vi "simulation_data.vi"() -> ()   [LabVIEW 2024]
uses:
  <vilib>/Utility/file.llb/Read Delimited Spreadsheet (string).vi
  <vilib>/ptbypt/NI_PtbyPt.lvlib
panel:
  out "double precision float":dbl
  out "XY Graph":cluster{dbl[], dbl[]}[](graph)
  in  "stop":bool
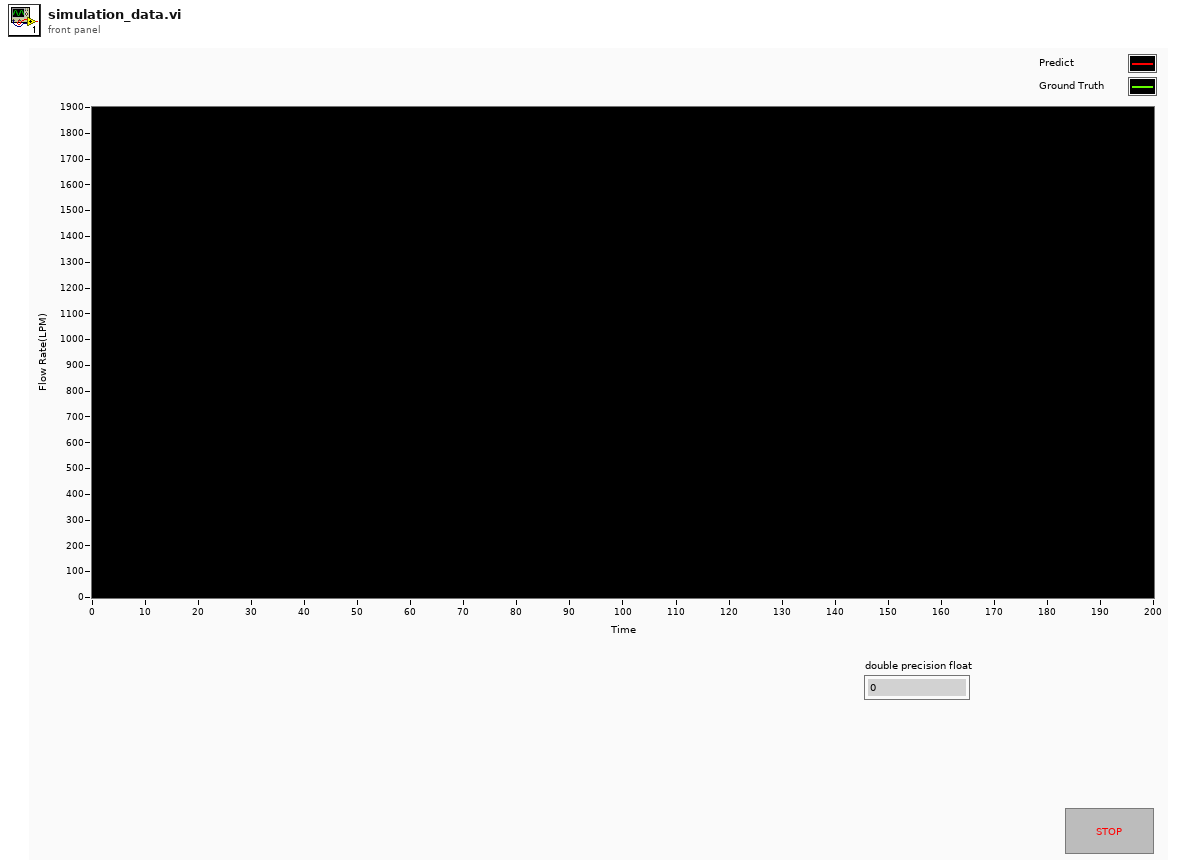
[diagram p1: front panel]
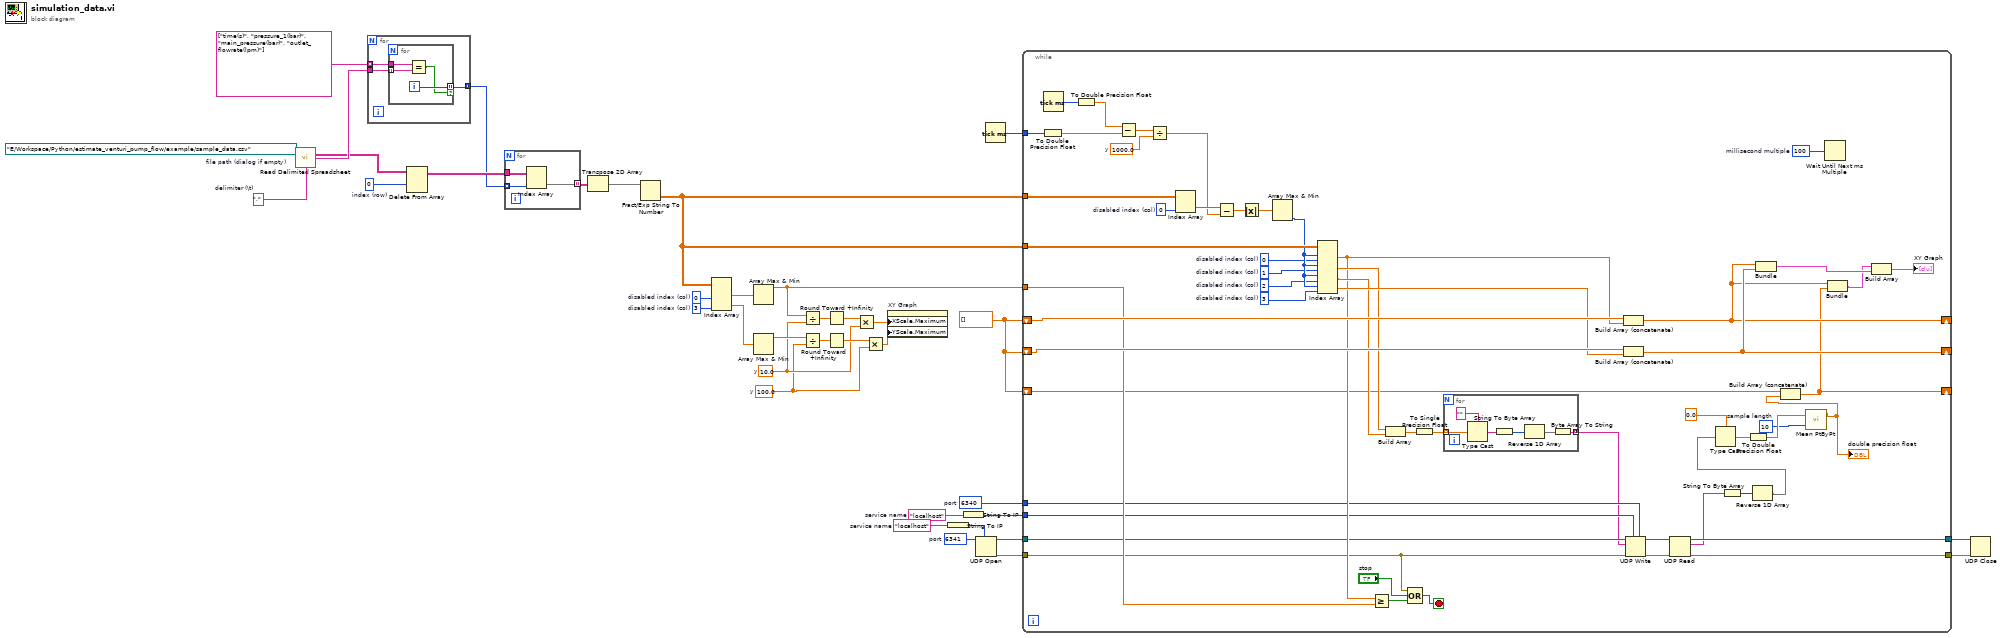
[diagram p0: block diagram]
diagram:
  w5 = "localhost"  # service name
  w1 = u16 6340  # port
  w8 = "localhost"  # service name
  w7 = u16 6341  # port
  w13 = 100.0  # y
  w16 = 10.0  # y
  w9 = dbl[] []
  w24 = 3  # disabled index (col)
  w25 = 0  # disabled index (col)
  w32 = 0  # index (row)
  w36 = ","  # delimiter (\t)
  w37 = path "E:/Workspace/Python/estimate_venturi_pump_flow/example/sample_data.csv"  # file path (dialog if empty)
  n1 = call-poly <vilib>:"Read Delimited Spreadsheet.vi"("file path (dialog if empty)"=w37, "delimiter (\\t)"=w36) -> ("all rows"=w33:string[][], "first row"=w35:string[])  [unwired: 8 in, 4 out]
  n2 = for {
    tunnel: w35 -> [w40]
    tunnel: string[] ["time(s)", "pressure_1(bar)", "main_pressure(bar)", "outlet_flowrate(lpm)"] -> [w39] mode=indexing
    tunnel: [w38] -> w30 mode=concatenating
    n3 = for {
      tunnel: w40 -> [w44] mode=indexing
      tunnel: w39 -> [w43]
      tunnel: [w42] -> w38 mode=indexing if=w41
      i -> [w42]
      n4 = Equal?(x=w43, y=w44) -> (x = y?=w41:bool)
    }
  }
  n5 = Delete From Array "Delete From Array"(array=w33, index (row)=w32) -> (array with subset deleted=w31:string[][])  [unwired: 2 in, 1 out]
  n6 = for {
    tunnel: w31 -> [w47]
    tunnel: w30 -> [w46] mode=indexing
    tunnel: [w45] -> w29 mode=indexing
    n7 = Index Array "Index Array"(array=w47, index (col)=w46) -> (element=w45:string[])  [unwired: 1 in]
  }
  n8 = Transpose 2D Array(2D array=w29) -> (transposed array=w28:string[][])
  n9 = Fract/Exp String To Number(string=w28) -> (number=w26:dbl[][])  [unwired: 3 in, 1 out]
  n10 = Index Array "Index Array"(array=w26, index (col) #1=w25, index (col) #2=w24) -> (element #1=w23:dbl[], element #2=w22:dbl[])  [unwired: 2 in]
  n11 = Array Max & Min(array=w23) -> (max value=w12:dbl)  [unwired: 3 out]
  n12 = Array Max & Min(array=w22) -> (max value=w21:dbl)  [unwired: 3 out]
  n13 = Divide(x=w12, y=w16) -> (x/y=w20:dbl)
  n14 = Divide(x=w21, y=w13) -> (x/y=w19:dbl)
  n15 = Round Toward +Infinity(x=w20) -> (ceil(x): smallest int >= x=w18:dbl)
  n16 = Round Toward +Infinity(x=w19) -> (ceil(x): smallest int >= x=w17:dbl)
  n17 = Multiply(x=w18, y=w16) -> (x*y=w15:dbl)
  n18 = Multiply(x=w17, y=w13) -> (x*y=w14:dbl)
  n19 = property on="XY Graph" class="XYGraph (strict)"("XScale.Maximum"=w15, "YScale.Maximum"=w14) -> ()  [unwired: 2 in, 2 out]
  n20 = String To IP(1:w8) -> (0:w6:u32)
  n21 = String To IP(1:w5) -> (0:w2:u32)
  n22 = UDP Open(7:w6, 11:w7) -> (port=w4:refnum<k16>, 0:w3:errorcluster)  [unwired: 3 in, 1 out]
  n23 = Tick Count (ms)() -> (millisecond timer value=w27:u32)
  n24 = while {
    tunnel: w27 -> [w100]
    tunnel: w26 -> [w95]
    tunnel: w26 -> [w89]
    shift-right: [w66] -> _
    shift-left: w9 -> [w82]
    shift-right: [w67] -> _
    shift-left: w9 -> [w81]
    tunnel: w12 -> [w73]
    tunnel: w4 -> [w71]
    tunnel: w3 -> [w56]
    tunnel: [w62] -> w11
    tunnel: [w61] -> w10
    shift-right: [w65] -> _
    shift-left: w9 -> [w69]
    tunnel: w2 -> [w58]
    tunnel: w1 -> [w57]
    stop <- w75 stop-if-true
    w49 = 10  # sample length
    w83 = 3  # disabled index (col)
    w84 = 2  # disabled index (col)
    w85 = 1  # disabled index (col)
    w86 = 0  # disabled index (col)
    w94 = 0  # disabled index (col)
    w96 = 1000.0  # y
    w102 = u32 100  # millisecond multiple
    n25 = To Double Precision Float(number=w100) -> (double precision float=w98:dbl)
    n26 = Tick Count (ms)() -> (millisecond timer value=w101:u32)
    n27 = To Double Precision Float(number=w101) -> (double precision float=w97:dbl)
    n28 = Subtract(x=w97, y=w98) -> (x-y=w99:dbl)
    n29 = Divide(x=w99, y=w96) -> (x/y=w92:dbl)
    n30 = Index Array "Index Array"(array=w95, index (col)=w94) -> (element=w93:dbl[])  [unwired: 1 in]
    n31 = Subtract(x=w93, y=w92) -> (x-y=w91:dbl[])
    n32 = Absolute Value(x=w91) -> (abs(x)=w90:dbl[])
    n33 = Array Max & Min(array=w90) -> (min index (indices)=w88:i32)  [unwired: 3 out]
    n34 = Index Array "Index Array"(array=w89, index (row) #1=w88, index (col) #1=w86, index (row) #2=w88, index (col) #2=w85, index (row) #3=w88, index (col) #3=w84, index (row) #4=w88, index (col) #4=w83) -> (element #1=w74:dbl, element #2=w78:dbl, element #3=w77:dbl, element #4=w80:dbl)
    n35 = Greater Or Equal?(x=w74, y=w73) -> (x >= y?=w72:bool)
    n36 = Build Array "Build Array"(w78, w77) -> (w76:dbl[])
    n37 = Compound Arithmetic op=OR(w56, "stop", w72) -> (w75:bool)
    n38 = To Single Precision Float(number=w76) -> (single precision float=w55:sgl[])
    n39 = for {
      tunnel: w55 -> [w108] mode=indexing
      tunnel: [w103] -> w54 mode=concatenating
      n40 = Type Cast(type="" ("data out"), x=w108) -> (*(type *) &x=w106:string)
      n41 = String To Byte Array(string=w106) -> (unsigned byte array=w105:u8[])
      n42 = Reverse 1D Array(array=w105) -> (reversed array=w104:u8[])
      n43 = Byte Array To String(unsigned byte array=w104) -> (string=w103:string)
    }
    n44 = Build Array (concatenate)(w82, w74) -> (w66:dbl[])
    n45 = Build Array (concatenate)(w81, w80) -> (w67:dbl[])
    n46 = UDP Write(address=w58, port or service name=w57, connection ID=w71, data in=w54, 8:w56) -> (error out=w59:errorcluster, 3:w60:refnum<k16>)  [unwired: 1 in]
    n47 = UDP Read(connection ID=w60, 8:w59) -> (data out=w53:string, error out=w61:errorcluster, 3:w62:refnum<k16>)  [unwired: 2 in, 2 out]
    n48 = String To Byte Array(string=w53) -> (unsigned byte array=w52:u8[])
    n49 = Reverse 1D Array(array=w52) -> (reversed array=w51:u8[])
    n50 = Type Cast(type=sgl 0.0 ("String"), x=w51) -> (*(type *) &x=w68:sgl)
    n51 = To Double Precision Float(number=w68) -> (double precision float=w50:dbl)
    n52 = Bundle(w66, w67) -> (w79:cluster{dbl[], dbl[]})  [unwired: 1 in]
    n53 = call <vilib>:"Mean PtByPt.vi"("x"=w50, "sample length"=w49) -> ("mean"=w48:dbl)  [unwired: 2 in, 1 out]
    "double precision float" <- w48
    n54 = Build Array (concatenate)(w69, w48) -> (w65:dbl[])
    n55 = Wait Until Next ms Multiple(millisecond multiple=w102) -> ()  [unwired: 1 out]
    n56 = Bundle(w66, w65) -> (w63:cluster{dbl[], dbl[]})  [unwired: 1 in]
    n57 = Build Array(w63, w79) -> (→"XY Graph":cluster{dbl[], dbl[]}[])
  }
  n58 = UDP Close(connection ID=w11, 8:w10) -> ()  [unwired: 2 out]
